vi "Integral Compensator.vi"() -> ()   [LabVIEW 2020]
uses:
  <vilib>/MakerHub/LINX/Public/Peripherals/Analog/Analog Read 1 Chan.vi
  <vilib>/MakerHub/LINX/Private/Local IO/LinxI2cWrite.vi
  <vilib>/MakerHub/LINX/Public/Utilities/Check Channel.vi
  <vilib>/MakerHub/LINX/Public/Peripherals/Analog/Analog Read N Chans.vi
  <vilib>/MakerHub/LINX/Private/Local IO/LinxAnalogRead.vi
  <vilib>/MakerHub/LINX/Public/Utilities/Open Serial.vi
  <vilib>/MakerHub/LINX/Private/Utilties/Generate Error.vi
  <vilib>/MakerHub/LINX/LMH-LINX.lvlib
panel:
  out "Salida":dynamicdata(graph)
  out "Señal de control":dbl(graph)
  out "r":dbl
  out "T":dbl
  out "IT":i32
  in  "SET":bool
  in  "Ref":dbl(slide) min=0.0 max=5.0 step=0.5 scale=0.0..5.0
  out "Error":dbl(graph)
  in  "tsim":dbl
  # "U(z)\n----\nE(z)"
  # "0.03515 z^2 + 0.003242 z - 0.03191\n  ----------------------------------\n        z^2 - 1.824 z + 0.8237"
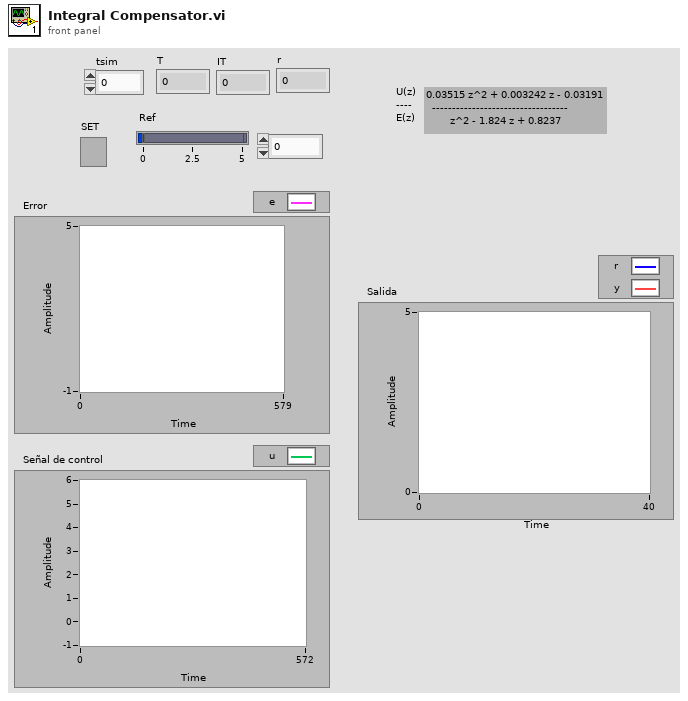
[diagram p1: front panel]
types:
  T1 = typedef "LMH-LINX.lvlib/LINX Ref.ctl" = cluster{"IO":T2, "Interface":T3, "LINX Device Config":T4}
  T2 = typedef "LMH-LINX.lvlib/Platform.ctl" = enum16{"Remote", "Local"}
  T3 = typedef "LMH-LINX.lvlib/Interface.ctl" = enum16{"Serial", "TCP"}
  T4 = typedef "LMH-LINX.lvlib/Device.lvlib/LINX Device Config.ctl" = cluster{"Interface":T3, "COM Port":refnum<visa-resource-name>, "TCP Configuration":T5, "Device Family":u8, "Device ID":u8, "Device Name":string, "TCP Ref":refnum<k5>, "Channels":T6}
  T5 = typedef "LMH-LINX.lvlib/Device.lvlib/TCP Config.ctl" = cluster{"IP Address":string, "Port":u16}
  T6 = typedef "LMH-LINX.lvlib/Channels.ctl" = cluster{"DI":u8[], "DO":u8[], "AI":u8[], "AO":u8[], "PWM":u8[], "QE":u8[], "UART":u8[], "I2C 2":u8[], "SPI":u8[], "CAN":u8[], "Servo":u8[], "AI Ref (V)":dbl, "AI Resolution (Bits)":u8, "AO Ref (V)":dbl, "AO Resolution (Bits)":u8}
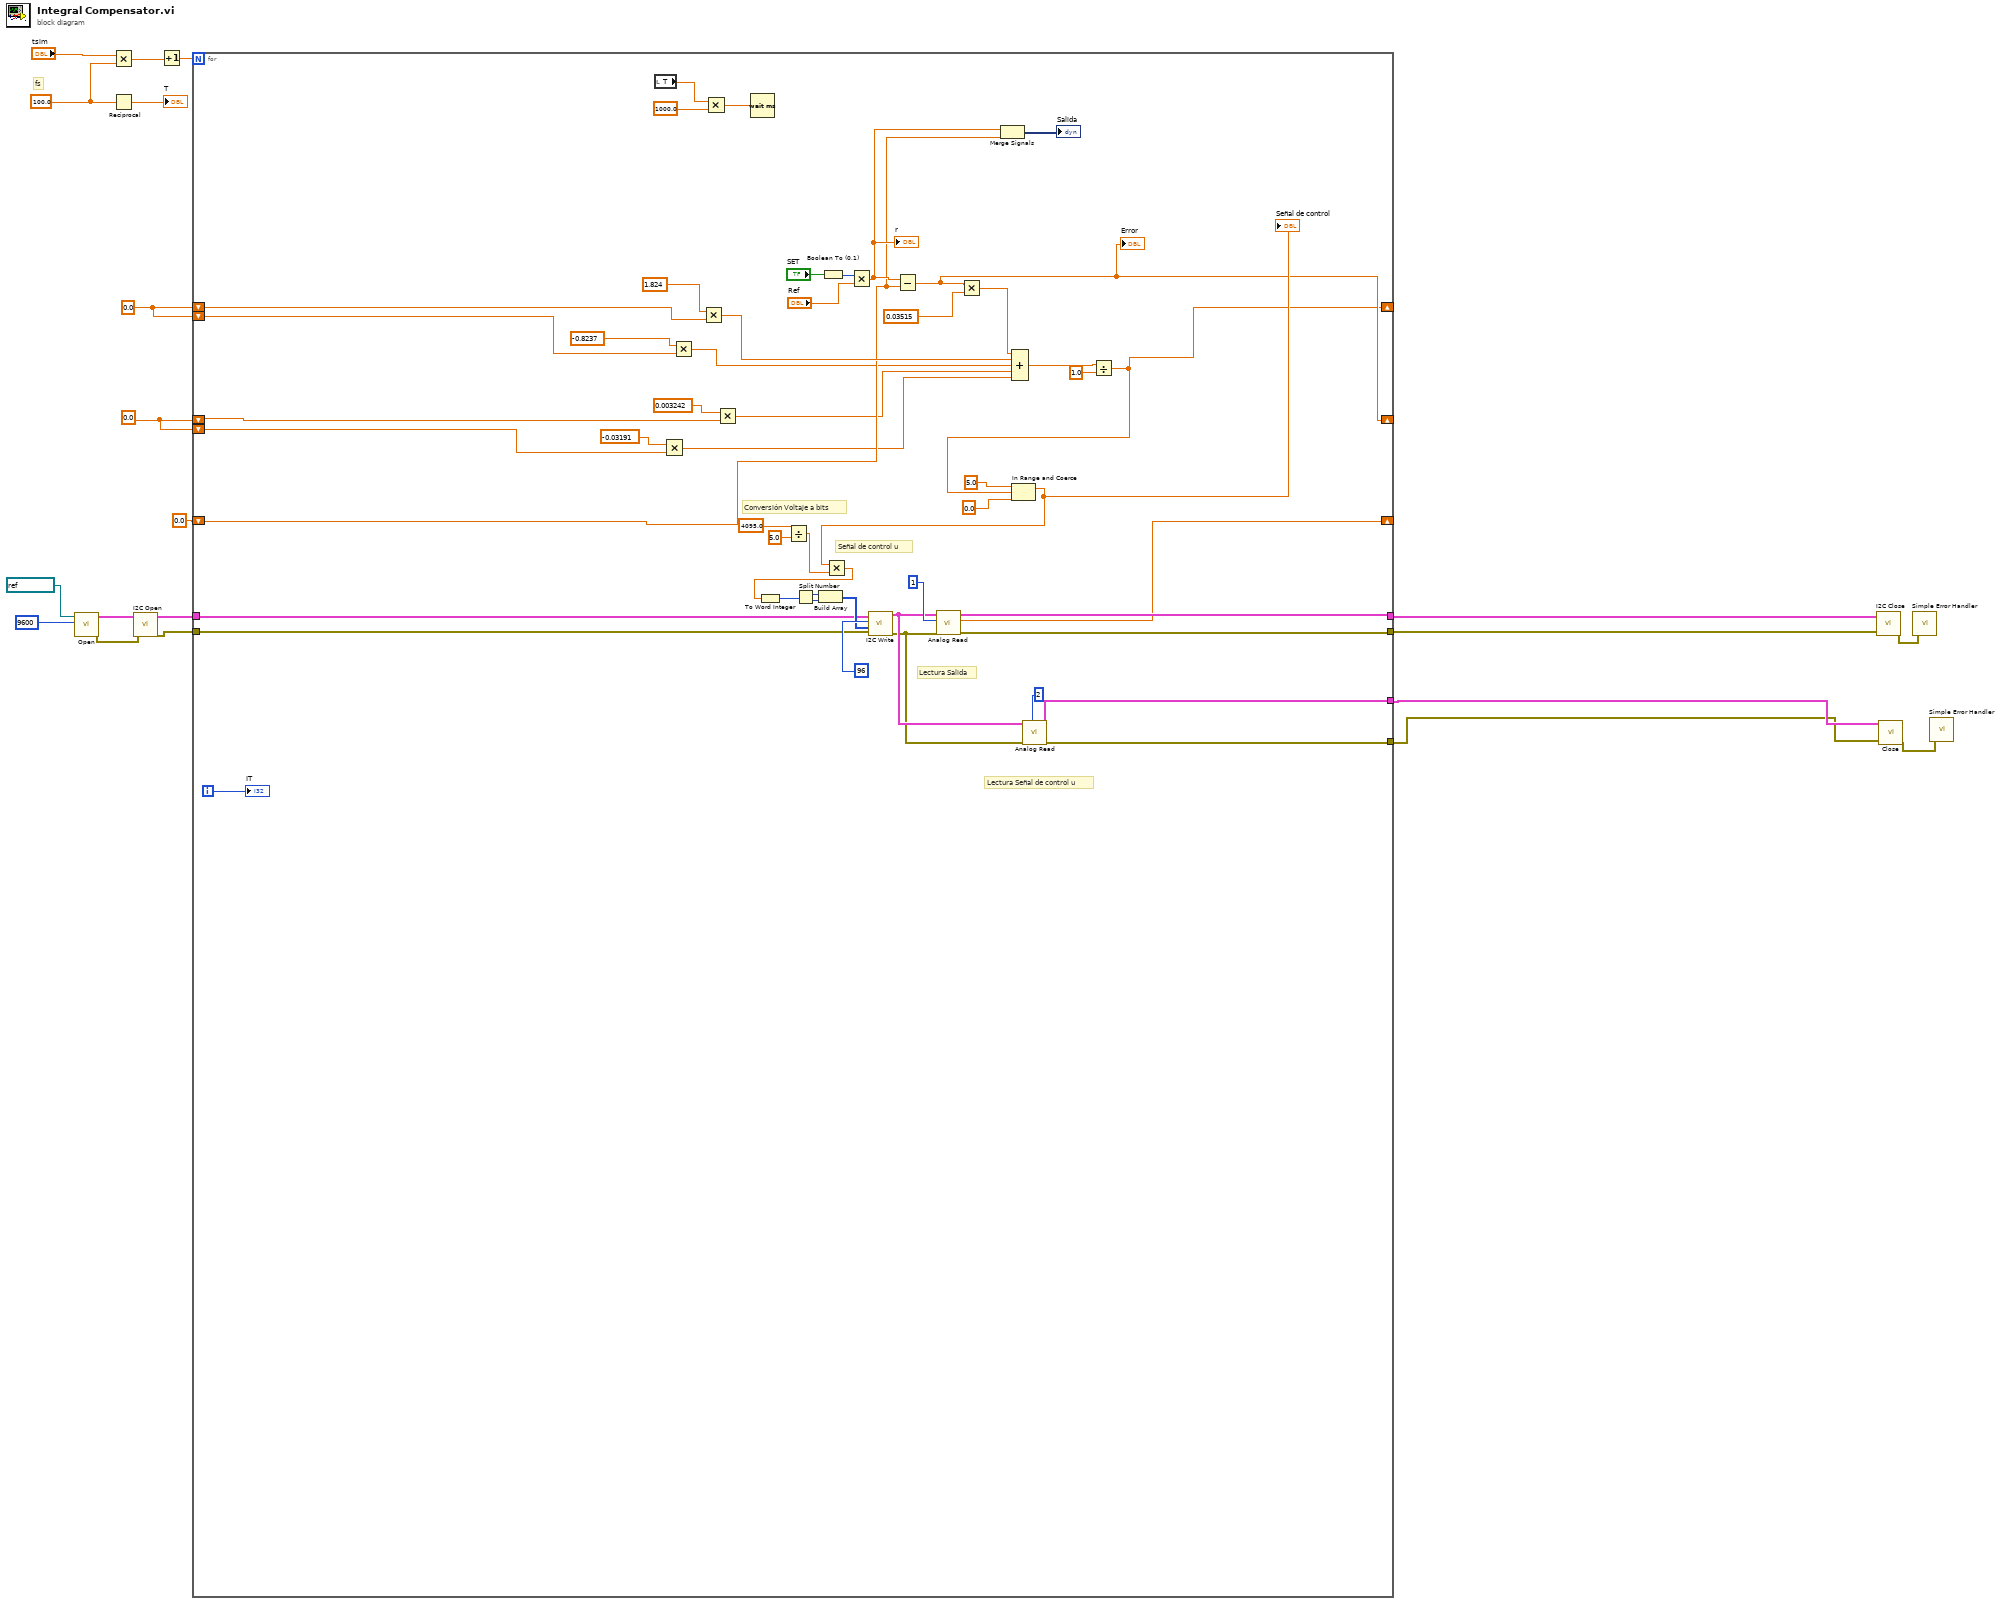
[diagram p0: block diagram]
diagram:
  w1 = 0.0
  w17 = 100.0 ("y")
  w2 = 0.0
  # "fs"
  n1 = call-poly <vilib>:"Open.vi"("Baud Rate Override"=u32 9600, "Serial Port"=refnum<visa-resource-name> "COM5") -> ("Error Out"=w12:errorcluster, "LINX Resource"=w13:T1)  [unwired: 7 in, 1 out]
  n2 = Multiply(x="tsim", y=w17) -> (x*y=w20:dbl)
  n3 = Reciprocal(x=w17) -> (1/x=→"T":dbl)
  n4 = call <vilib>:"I2C Open.vi"("Error In"=w12, "LINX Resource"=w13) -> ("Error Out"=w5:errorcluster, "LINX Resource"=w6:T1)  [unwired: 8 in]
  n5 = Increment(x=w20) -> (x+1=w19:dbl)
  n6 = for {
    N: w19 -> [_]
    shift-right: [w28] -> _
    shift-left: w1 -> [w36]
    shift-right: [w30] -> _
    shift-left: w2 -> [w41]
    shift-right: [w40] -> _
    shift-left: 0.0 ("Voltage") -> [w39]
    tunnel: w6 -> [w38]
    tunnel: [w45] -> w10
    tunnel: w5 -> [w37]
    tunnel: [w44] -> w9
    tunnel: [w32] -> w4
    tunnel: [w31] -> w3
    shift-left: w2 -> [w26]
    shift-left: w1 -> [w24]
    i -> [w68]
    # "Conversión Voltaje a bits"
    # "Señal de control u"
    # "Lectura Señal de control u"
    # "Lectura Salida"
    n7 = local read "T"() -> (w71:dbl)
    n8 = Multiply(x=-0.03191, y=w26) -> (x*y=w23:dbl)
    n9 = Multiply(x=-0.8237, y=w24) -> (x*y=w21:dbl)
    n10 = Multiply(x=1.824, y=w36) -> (x*y=w61:dbl)
    n11 = Multiply(x=w71, y=1000.0) -> (x*y=w69:dbl)
    n12 = Multiply(x=0.003242, y=w41) -> (x*y=w22:dbl)
    n13 = Wait (ms)(milliseconds to wait=w69) -> ()  [unwired: 1 out]
    n14 = Divide ("Divide 2")(x=4095.0 ("Constant"), y=5.0 ("y 2")) -> (x/y=w51:dbl)
    n15 = Boolean To (0,1)(Boolean="SET") -> (0, 1=w66:i16)
    n16 = Multiply(x=w66, y="Ref") -> (x*y=w43:dbl)
    "r" <- w43
    n17 = Subtract(x=w43, y=w39) -> (x-y=w30:dbl)
    "Error" <- w30
    n18 = Multiply(x=w30, y=0.03515) -> (x*y=w29:dbl)
    n19 = Merge Signals(w43, w39) -> (→"Salida":dynamicdata)
    n20 = Compound Arithmetic op=ADD(w29, w61, w21, w22, w23) -> (w60:dbl)
    n21 = Divide(x=w60, y=1.0) -> (x/y=w28:dbl)
    n22 = In Range and Coerce(upper limit=5.0, x=w28, lower limit=0.0) -> (coerced(x)=w33:dbl)  [unwired: 1 out]
    "Señal de control" <- w33
    n23 = Multiply(x=w33, y=w51) -> (x*y=w50:dbl)
    n24 = To Word Integer(number=w50) -> (16bit integer=w54:i16)
    n25 = Split Number(x=w54) -> (hi(x)=w53:u8, lo(x)=w52:u8)
    n26 = Build Array ("Build Array 4")(w53, w52) -> (w49:u8[])
    n27 = call <vilib>:"I2C Write.vi"("Error In"=w37, "Data"=w49, "I2C Slave Address (0)"=u8 96, "LINX Resource"=w38) -> ("Error Out"=w46:errorcluster, "LINX Resource"=w47:T1)  [unwired: 6 in]
    n28 = call-poly <vilib>:"Analog Read.vi"("Error In"=w46, "Analog Channel"=u8 1 ("AO Channel"), "LINX Resource"=w47) -> ("Error Out"=w44:errorcluster, "Voltage"=w40:dbl, "LINX Resource"=w45:T1)  [unwired: 5 in, 1 out]
    n29 = call-poly <vilib>:"Analog Read.vi"("Error In"=w46, "Analog Channel"=u8 2, "LINX Resource"=w47) -> ("Error Out"=w31:errorcluster, "LINX Resource"=w32:T1)  [unwired: 5 in, 2 out]
    "IT" <- w68
  }
  n30 = call <vilib>:"I2C Close.vi"("Error In"=w9, "LINX Resource"=w10) -> ("Error Out"=w11:errorcluster)  [unwired: 8 in, 1 out]
  n31 = call <vilib>:"Close.vi"("Error In"=w3, "LINX Resource"=w4) -> ("Error Out"=w8:errorcluster)  [unwired: 9 in]
  n32 = call <vilib>:"Simple Error Handler.vi"("error in (no error)"=w11) -> ()  [unwired: 4 in, 5 out]
  n33 = call <vilib>:"Simple Error Handler.vi"("error in (no error)"=w8) -> ()  [unwired: 4 in, 5 out]
